vi "Report_Do.vi"(9 "Array":refnum<class "Report Data.lvclass">[](array[class]), 10 "Action Data":T1, 11 "Report Handler in":refnum<class "Report Handler.lvclass">) -> (0 "error out":errorcluster)   [LabVIEW 2020, in "ProjectBuilder.lvlib" / "Report Handler.lvclass"]
uses:
  Report Handler.lvclass
  Ctl/Ctl_Action Data.ctl
  ProjectBuilder.lvlib
  Report Data/Report Data.lvclass
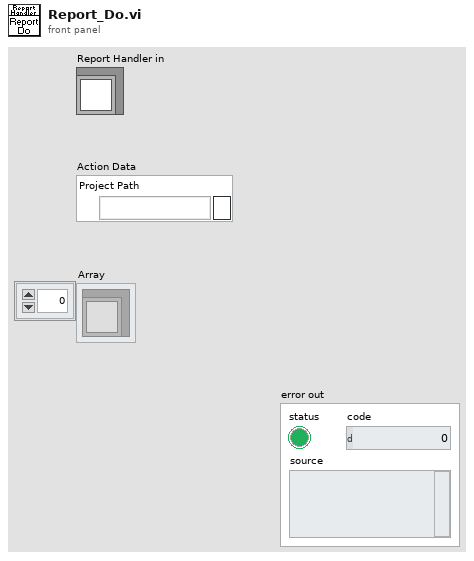
[diagram p1: front panel]
types:
  T1 = typedef "ProjectBuilder.lvlib/Ctl_Action Data.ctl" = cluster{"Project Path":path}
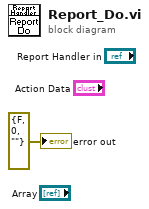
[diagram p0: block diagram]
diagram:
  "error out" <- errorcluster {"status"=FALSE, "code"=0, "source"=""} ("error in (no error)")
